vi "GetForceCalibParams2.vi"(4 "error in (no error)":errorcluster, 5 "F0 (pN)":dbl=0.01 caption="F min (pN)" format="%#g", 6 "L1 (mm)":dbl=1.4 caption="F max (pN)" format="%#g", 7 "Fmax (pN)":dbl=85.0 caption="Decay length (mm)" format="%#g") -> (0 "error out":errorcluster, 1 "F1/L1/F0/F2/L2":dbl[](array[numeric])=[49.0, 1.45, 0.01, 21.000000000000004, 0.6])   [LabVIEW 2018]
doc: "Displays a standard dialog box that prompts users to enter information, such as a user name and password.\n--------------------\n\nThis Express VI is configured as follows:\n\nMessage to Display to the User:Magnet/bead parameters\nThe inputs are: \nNumber: Decay length (mm)\nNumber: F max (pN)\nNumber: F min (pN)"
panel:
  in  "Cancel":bool caption="OK1"
  in  "F1/Fmax":dbl=0.7 caption="Decay length (mm)" format="%#g"
  in  "L2 (mm)":dbl=0.8 caption="F max (pN)" format="%#g"
  out "Fmax/decay/Fmin":dbl[](array[numeric])=[70.0, 1.45, 0.01]
  out "F min (pN)":dbl=0.01 format="%#g"
  out "Decaylength (mm)":dbl=1.45 caption="F max (pN)" format="%#g"
  out "F max (pN)":dbl=70.0 caption="Decay length (mm)" format="%#g"
  out "OK":bool=TRUE
  in  "OK1":bool
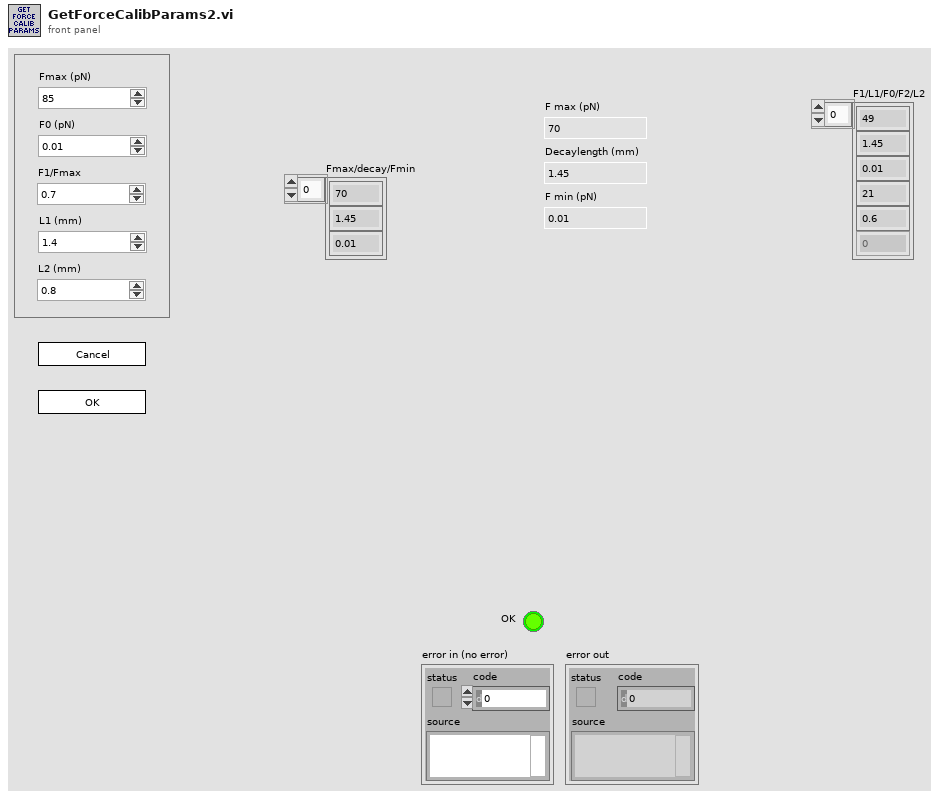
[diagram p1: front panel]
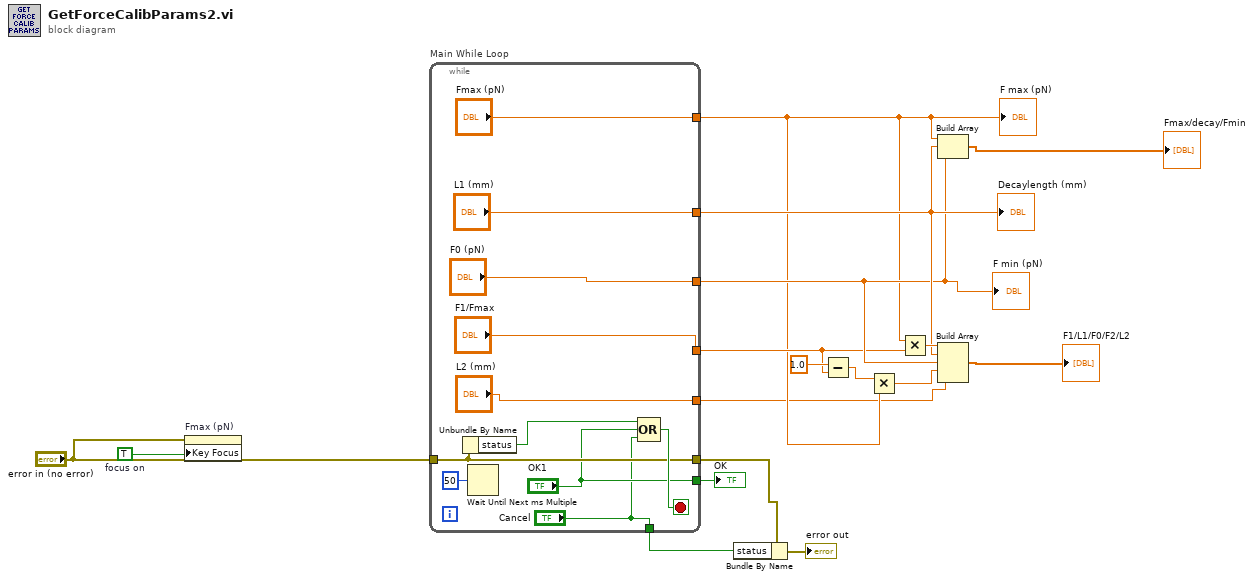
[diagram p0: block diagram]
diagram:
  w16 = TRUE  # focus on
  n1 = property on="Fmax (pN)" class="DigNum (strict)"(error in="error in (no error)", "Key Focus"=w16) -> ()  [unwired: 1 in, 2 out]
  n2 = while "Main While Loop" {
    tunnel: ["OK1"] -> w17
    tunnel: "error in (no error)" -> [w26]
    tunnel: [w26] -> w3
    tunnel: ["Fmax (pN)"] -> w7
    tunnel: ["L1 (mm)"] -> w12
    tunnel: ["F0 (pN)"] -> w11
    tunnel: ["F1/Fmax"] -> w9
    tunnel: ["L2 (mm)"] -> w5
    tunnel: ["Cancel"] -> w2
    stop <- w27 stop-if-true
    n3 = Unbundle By Name(w26) -> ("status"=w25:bool)
    n4 = Wait Until Next ms Multiple(millisecond multiple=u32 50) -> ()  [unwired: 1 out]
    n5 = Compound Arithmetic op=OR(w25, "OK1", "Cancel") -> (w27:bool)
  }
  "OK" <- w17
  "F max (pN)" <- w7
  "Decaylength (mm)" <- w12
  "F min (pN)" <- w11
  n6 = Bundle By Name(cluster=w3, "status"=w2) -> (→"error out":errorcluster)
  n7 = Subtract(x=1.0, y=w9) -> (x-y=w8:dbl)
  n8 = Multiply(x=w8, y=w7) -> (x*y=w6:dbl)
  n9 = Multiply(x=w7, y=w9) -> (x*y=w13:dbl)
  n10 = Build Array(w7, w12, w11) -> (→"Fmax/decay/Fmin":dbl[])
  n11 = Build Array(w13, w12, w11, w6, w5) -> (→"F1/L1/F0/F2/L2":dbl[])
